vi "CreateImageFromFonts.vi"() -> ()   [LabVIEW 2023]
panel:
  out "error out":errorcluster
  in  "error in (no error)":errorcluster
  out "text 3":string="Dt=                  1/Dt=\nD  =                 D   /Dt="
  out "text 2":string="Dt=                  1/Dt=\nD  =                 D   /Dt="
  out "text":string="Dt=                  1/Dt=\nD  =                 D   /Dt="
  out "With Numbers":picture
  out "No Numbers":picture
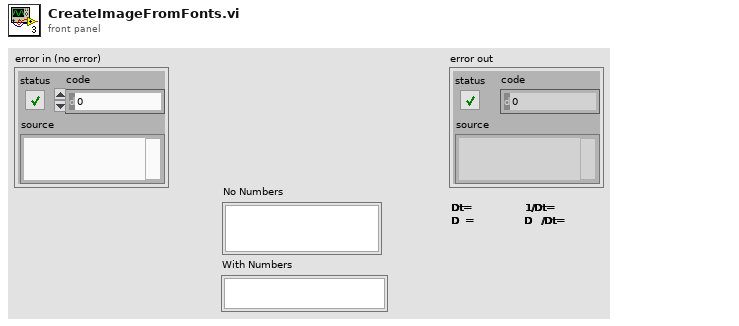
[diagram p1: front panel]
types:
  T1 = cluster{"Font Name:":string, "Size":i16, "Strikeout?":bool, "Italic?":bool, "Underline?":bool, "Outline?":bool, "Shadow?":bool, "Bold?":bool}
  T2 = enum16{"User-specified Font", "Application Font", "System Font", "Dialog Font"}
  T3 = cluster{"horizontal":enum16{"left", "center", "right"}, "vertical":enum16{"top", "center", "bottom"}}
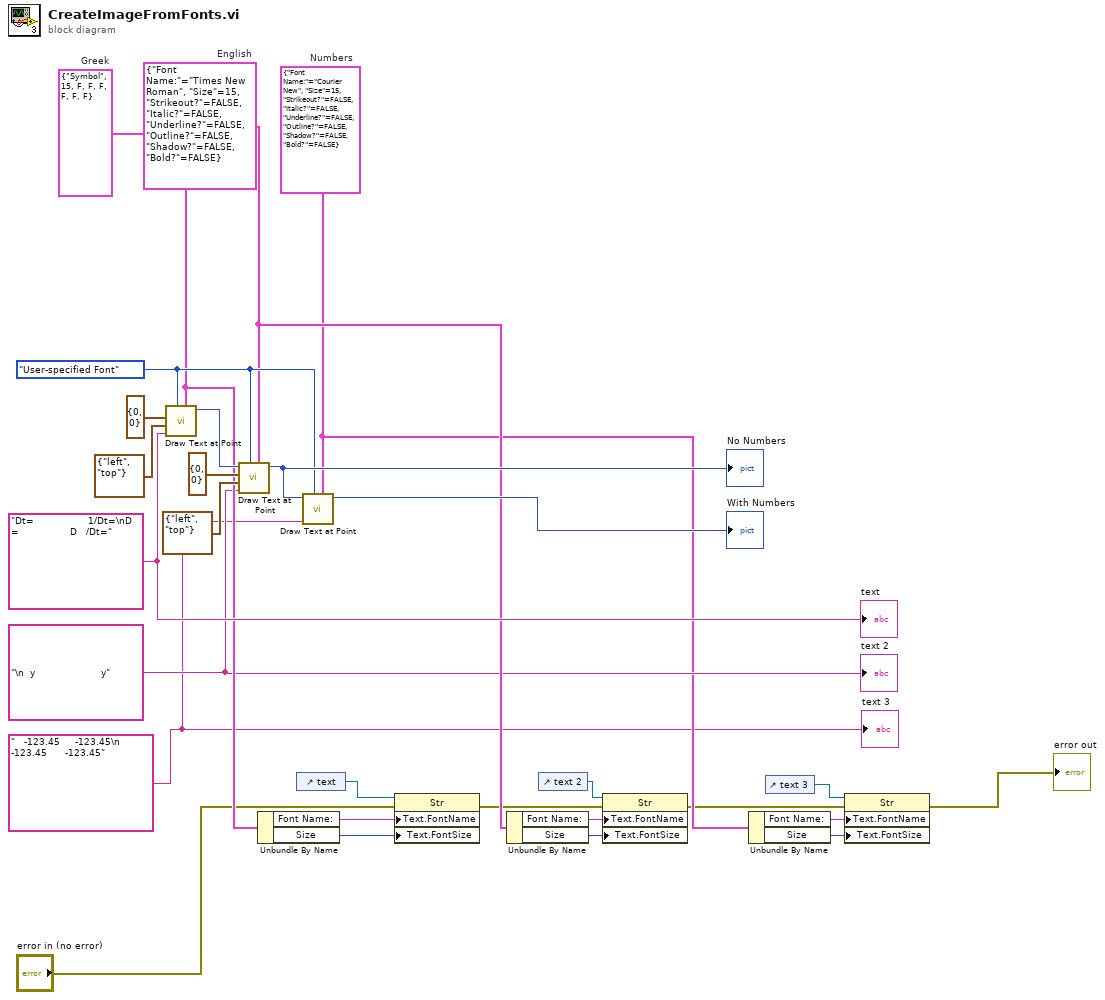
[diagram p0: block diagram]
diagram:
  w5 = "   -123.45     -123.45\n   -123.45      -123.45" ("text")
  w7 = T1 {"Font Name:"="Courier New", "Size"=15, "Strikeout?"=FALSE, "Italic?"=FALSE, "Underline?"=FALSE, "Outline?"=FALSE, "Shadow?"=FALSE, "Bold?"=FALSE}  # Numbers
  w20 = T2."User-specified Font" ("desired font(Application)")
  w10 = "\n  y                      y" ("text")
  w11 = T1 {"Font Name:"="Times New Roman", "Size"=15, "Strikeout?"=FALSE, "Italic?"=FALSE, "Underline?"=FALSE, "Outline?"=FALSE, "Shadow?"=FALSE, "Bold?"=FALSE}  # English
  w25 = "Dt=                  1/Dt=\nD  =                 D   /Dt=" ("text")
  w17 = T1 {"Font Name:"="Symbol", "Size"=15, "Strikeout?"=FALSE, "Italic?"=FALSE, "Underline?"=FALSE, "Outline?"=FALSE, "Shadow?"=FALSE, "Bold?"=FALSE}  # Greek
  n1 = call <vilib>:"Draw Text at Point.vi"("[user-specified font]"=w17, "desired font(Application)"=w20, "text"=w25, "alignment(left, top)"=T3 {"horizontal"=enum."left", "vertical"=enum."top"}, "origin"=cluster{"x":i16, "y":i16} {"x"=0, "y"=0}) -> ("new picture"=w22:picture)  [unwired: 5 in, 1 out]
  n2 = call <vilib>:"Draw Text at Point.vi"("[user-specified font]"=w11, "desired font(Application)"=w20, "text"=w10, "alignment(left, top)"=T3 {"horizontal"=enum."left", "vertical"=enum."top"}, "origin"=cluster{"x":i16, "y":i16} {"x"=0, "y"=0}, "picture"=w22) -> ("new picture"=w21:picture)  [unwired: 4 in, 1 out]
  "No Numbers" <- w21
  n3 = Unbundle By Name(w17) -> ("Font Name:"=w16:string, "Size"=w15:i16)
  n4 = control-ref of="text"() -> (w18:refnum<vi>)
  n5 = call <vilib>:"Draw Text at Point.vi"("[user-specified font]"=w7, "desired font(Application)"=w20, "text"=w5, "picture"=w21) -> ("new picture"=→"With Numbers":picture)  [unwired: 6 in, 1 out]
  n6 = property class="Str"(reference=w18, error in="error in (no error)", "Text.FontName"=w16, "Text.FontSize"=w15) -> (error out=w4:errorcluster)  [unwired: 1 out]
  n7 = Unbundle By Name(w11) -> ("Font Name:"=w13:string, "Size"=w12:i16)
  n8 = control-ref of="text 2"() -> (w14:refnum<vi>)
  n9 = property class="Str"(reference=w14, error in=w4, "Text.FontName"=w13, "Text.FontSize"=w12) -> (error out=w3:errorcluster)  [unwired: 1 out]
  n10 = Unbundle By Name(w7) -> ("Font Name:"=w9:string, "Size"=w8:i16)
  n11 = control-ref of="text 3"() -> (w6:refnum<vi>)
  n12 = property class="Str"(reference=w6, error in=w3, "Text.FontName"=w9, "Text.FontSize"=w8) -> (error out=→"error out":errorcluster)  [unwired: 1 out]
  "text" <- w25
  "text 2" <- w10
  "text 3" <- w5
